vi "VideoCapture GetBackendName.vi"(8 "error in (no error)":errorcluster, 11 "VideoCapture in":refnum<class "VideoCapture.lvclass">) -> (0 "error out":errorcluster, 2 "BackendName":string, 3 "VideoCapture out":refnum<class "VideoCapture.lvclass">)   [LabVIEW 2020, in "OpenLvVision_OpenCv.lvlib" / "VideoCapture.lvclass"]
doc: "Returns used backend API name."
uses:
  VideoCapture.lvclass
  C:/Users/lukas/Downloads/OpenLvVision_OpenCv/SourceCode/LabView/OpenLvVision_OpenCv/_LvHelpers/EdvrObject/EdvrObject.lvclass
  _LvHelpers/EdvrObject/EdvrObject.lvclass/EdvrObject.ctl
  OpenLvVision_OpenCv.lvlib
  _LvHelpers/EdvrObject/EdvrObject.lvclass
  Dlls/OlvOpenCvWrapper.dll
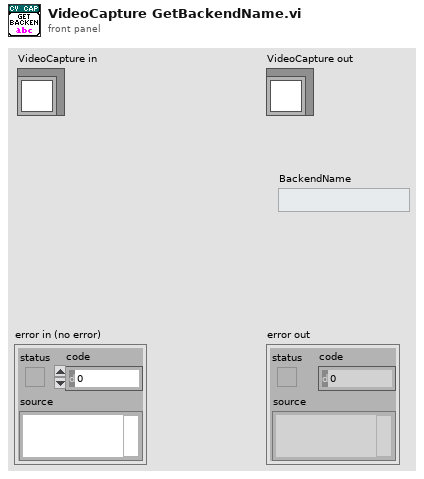
[diagram p1: front panel]
types:
  T1 = typedef "OpenLvVision_OpenCv.lvlib/EdvrObject.lvclass/Edvr.ctl" = refnum<data-value>
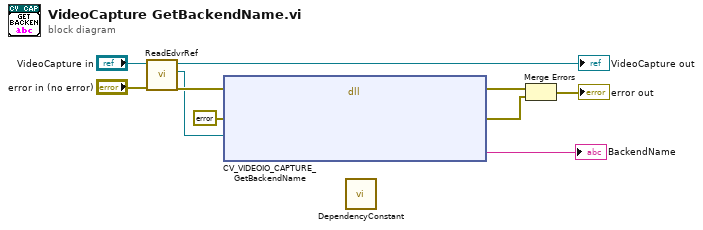
[diagram p0: block diagram]
diagram:
  n1 = call "ReadEdvrRef.vi"("error in (no error)"="error in (no error)", "EdvrObject in"="VideoCapture in") -> ("error out"=w8:errorcluster, "Edvr"=w7:T1, "EdvrObject out"=→"VideoCapture out":refnum<class "VideoCapture.lvclass">)  [unwired: 7 in]
  n2 = dll-call lib="C:/Users/lukas/Downloads/OpenLvVision_OpenCv/SourceCode/LabView/OpenLvVision_OpenCv/Dlls/OlvOpenCvWrapper.dll" fn="CV_VIDEOIO_CAPTURE_GetBackendName"(error in=w8, "Error"=errorcluster {"status"=FALSE, "code"=0, "source"=""} ("error out"), "edvrRef"=w7) -> (error out=w6:errorcluster, "Error"=w2:errorcluster, "resultHandle"=→"BackendName":string)  [unwired: 5 in, 1 out]
  n3 = call "DependencyConstant.vi"() -> ()  [unwired: 12 in]
  n4 = Merge Errors(w6, w2) -> (→"error out":errorcluster)
